vi "DP-Extract DPs and Noise.vi"(0 "state":T2, 1 "DP Freqs":T1, 5 "Mag":dbl[](array[numeric]) format="%.8f", 9 "Phase":dbl[](array[numeric]), 11 "SPL":dbl) -> (8 "Output Array":dbl[](array[numeric]))   [LabVIEW 2020]
uses:
  Typedefs/DP-Runtime State.ctl
  Typedefs/DP-Freqs.ctl
  c335da1f-e25d-4484-af00-f2f49c668875.vi
  0067a959-a5ee-42fc-8112-f8f00b49df11.vi
  db1ef7c5-0cc4-42b7-95b9-6f73bf8c4e9e.vi
  5d7fa8c8-6e1b-4af2-b079-9d590de1dffc.vi
  d56b4573-2391-4563-84da-4b5a0c978d84.vi
panel:
  # "SPL\nf1 (Hz)\nf2 (Hz)\nf1\nf2\n2f1-f2\nNse 2f1-f2\nf2-f1\nNse f2-f1\nPhase 2f1-f2"
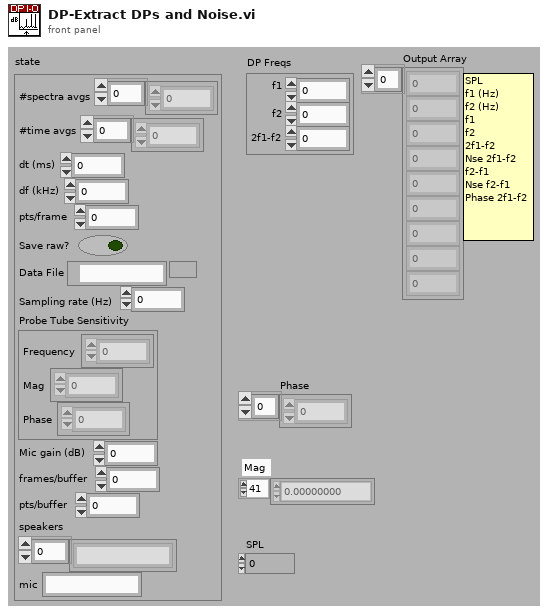
[diagram p1: front panel]
types:
  T1 = typedef "DP-Freqs.ctl" = cluster{"f1":dbl, "f2":dbl, "2f1-f2":dbl}
  T2 = typedef "DP-Runtime State.ctl" = cluster{"#spectra avgs":i32[], "#time avgs":i32[], "dt (ms)":dbl, "df (kHz)":dbl, "pts/frame":i32, "Save raw?":bool, "Data File":path, "Sampling rate (Hz)":dbl, "Probe Tube Sensitivity":cluster{"Frequency":dbl[], "Mag":dbl[], "Phase":dbl[]}, "Mic gain (dB)":dbl, "frames/buffer":i32, "pts/buffer":i32, "speakers":string[], "mic":string}
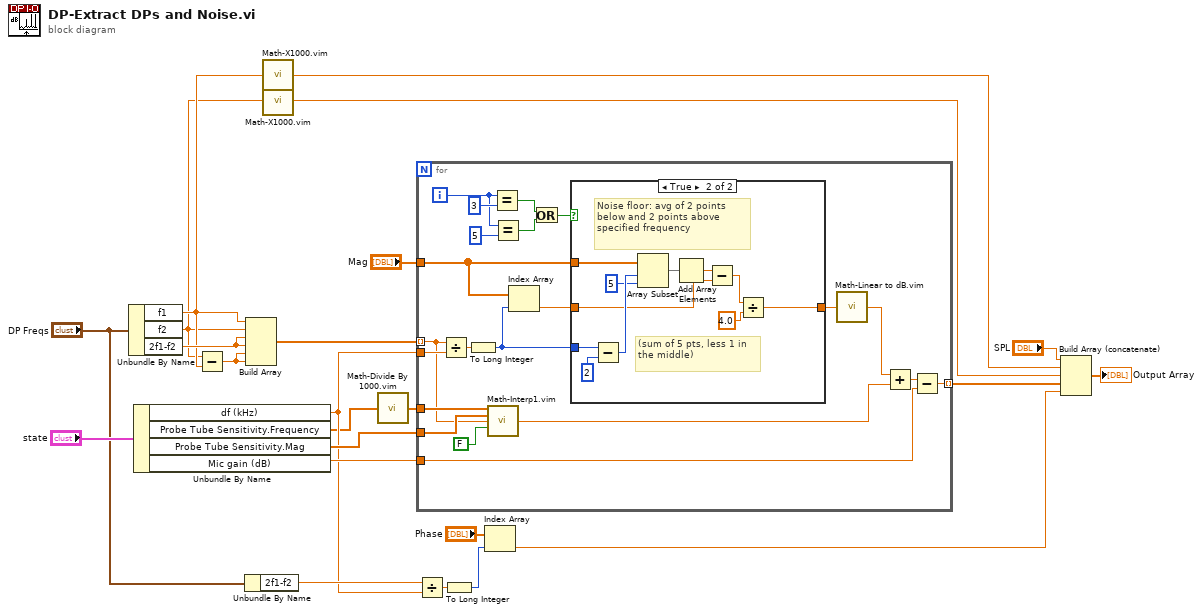
[diagram p0: block diagram]
diagram:
  n1 = Unbundle By Name("DP Freqs") -> ("f1"=w4:dbl, "f2"=w3:dbl, "2f1-f2"=w19:dbl)
  n2 = Unbundle By Name("state") -> ("df (kHz)"=w9:dbl, "Probe Tube Sensitivity.Frequency"=w1:dbl[], "Probe Tube Sensitivity.Mag"=w22:dbl[], "Mic gain (dB)"=w14:dbl)
  n3 = Subtract(x=w3, y=w4) -> (x-y=w18:dbl)
  n4 = Unbundle By Name("DP Freqs") -> ("2f1-f2"=w10:dbl)
  n5 = Build Array(w4, w3, w19, w19, w18, w18) -> (w17:dbl[])
  n6 = call "Math-X1000.vim"("X"=w4) -> ("1000X"=w6:dbl)
  n7 = call "Math-X1000.vim"("X"=w3) -> ("1000X"=w5:dbl)
  n8 = call "Math-Divide By 1000.vim"("X"=w1) -> ("1000X"=w2:dbl[])
  n9 = for {
    tunnel: w22 -> [w41]
    tunnel: [w44] -> w15 mode=indexing
    tunnel: w2 -> [w42]
    tunnel: w14 -> [w38]
    tunnel: w17 -> [w35] mode=indexing
    tunnel: "Mag" -> [w25]
    tunnel: w9 -> [w37]
    i -> [w33]
    n10 = Divide(x=w35, y=w37) -> (x/y=w36:dbl)
    n11 = To Long Integer(number=w36) -> (32bit integer=w27:i32)
    n12 = call "Math-Interp1.vim"("X"=w42, "Y"=w41, "U"=w35, "extrapolate (T)"=FALSE) -> ("V"=w39:dbl)  [unwired: 11 in]
    n13 = Equal?(x=w33, y=3) -> (x = y?=w30:bool)
    n14 = Equal?(x=w33, y=5) -> (x = y?=w29:bool)
    n15 = Index Array(array=w25, index=w27) -> (element=w28:dbl)
    n16 = Or(x=w30, y=w29) -> (x .or. y?=w31:bool)
    n17 = case shown="True" w31 {
      tunnel: w28 -> [w45 w51]
      tunnel: w27 -> [_ w56]
      tunnel: [w45 w46] -> w26
      tunnel: w25 -> [_ w47]
      frame False {
      }
      frame True {
        # "(sum of 5 pts, less 1 in the middle)"
        # "Noise floor: avg of 2 points\nbelow and 2 points above specified frequency"
        n18 = Subtract(x=w56, y=2) -> (x-y=w54:i32)
        n19 = Array Subset(array=w47, index=w54, length=5) -> (w52:dbl[])
        n20 = Add Array Elements(numeric array=w52) -> (sum=w48:dbl)
        n21 = Subtract(x=w48, y=w51) -> (x-y=w50:dbl)
        n22 = Divide(x=w50, y=4.0) -> (x/y=w46:dbl)
      }
    }
    n23 = call "Math-Linear to dB.vim"("linear"=w26) -> ("dB"=w40:dbl)
    n24 = Add(x=w40, y=w39) -> (x+y=w43:dbl)
    n25 = Subtract(x=w43, y=w38) -> (x-y=w44:dbl)
  }
  n26 = Divide(x=w10, y=w9) -> (x/y=w13:dbl)
  n27 = To Long Integer(number=w13) -> (32bit integer=w12:i32)
  n28 = Index Array(array="Phase", index=w12) -> (element=w7:dbl)
  n29 = Build Array (concatenate)("SPL", w6, w5, w15, w7) -> (→"Output Array":dbl[])
